vi "AddBufferEX_debug.vi"(0 "ph":u64, 5 "BuffNr":i16, 7 "1stImage":u32, 9 "LastImage":u32, 11 "error in (no error)":errorcluster, 12 "XRes":u16, 13 "YRes":u16, 14 "BitPerPixel":u16) -> (4 "hout":u64, 8 "ErrorCode":i32, 15 "error out":errorcluster)   [LabVIEW 2015]
doc: "Adds a buffer to the driver queue. This function returns immediately. If the desired image is transferred to the buffer a buffer event will be created.Once an event is created, the data can be retreived using GetImageBuffer.vi. This function is used to view images while the recording is enabled. To read out previously recorded images, use GetImageEx.vi."
uses:
  SC2_Cam.dll
panel:
  out "x-y":dbl
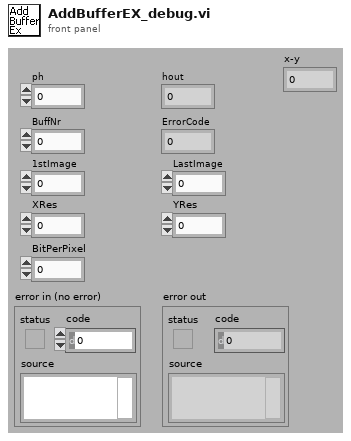
[diagram p1: front panel]
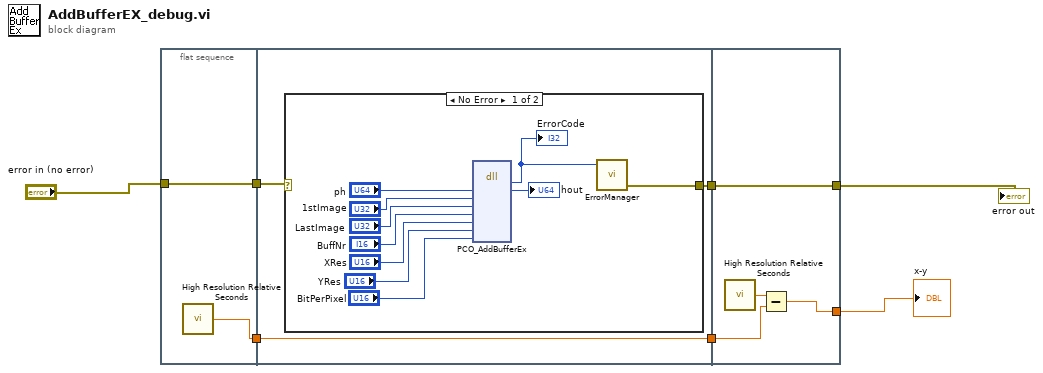
[diagram p0: block diagram]
diagram:
  n1 = flat-sequence {
    tunnel: "error in (no error)" -> [w9]
    tunnel: [w9] -> w5
    tunnel: [w8] -> w2
    tunnel: w5 -> [w12]
    tunnel: [w11] -> w4
    tunnel: [w10] -> w3
    tunnel: w2 -> [w10]
    tunnel: [w27] -> w6
    tunnel: w4 -> [w27]
    tunnel: w3 -> [w25]
    tunnel: [w24] -> w1
    frame #0 {
      n2 = call <vilib>:"High Resolution Relative Seconds.vi"() -> ("relative seconds"=w8:dbl)
    }
    frame #1 {
      n3 = case shown="No Error" w12 {
        selector: w12 -> [_ w23]
        tunnel: [w20 w23] -> w11
        frame No Error {
          n4 = dll-call lib="W:/Labview/Front ends/ARPEScontrol/subvi/PCO/32bit/SC2_Cam.dll" fn="PCO_AddBufferEx"("handle"="ph", "1stImage"="1stImage", "LastImage"="LastImage", "BuffNr"="BuffNr", "XRes"="XRes", "YRes"="YRes", "BitPerPixel"="BitPerPixel") -> ("return type"=w19:i32, "handle"=→"hout":u64)  [unwired: 9 in, 2 out]
          "ErrorCode" <- w19
          n5 = call "ErrorManager.vi"("ErrorCode"=w19) -> ("ErrorOut"=w20:errorcluster)  [unwired: 4 in]
        }
        frame Error {
        }
      }
    }
    frame #2 {
      n6 = call <vilib>:"High Resolution Relative Seconds.vi"() -> ("relative seconds"=w26:dbl)
      n7 = Subtract(x=w26, y=w25) -> (x-y=w24:dbl)
    }
  }
  "error out" <- w6
  "x-y" <- w1
